vi "laser control with polarimeter feedback.vi"() -> ()   [LabVIEW 2018]
uses:
  <vilib>/DAQmx/read.llb/DAQmx Read (Analog Wfm 1Chan NSamp).vi
  <vilib>/DAQmx/write.llb/DAQmx Write (Analog DBL 1Chan 1Samp).vi
  <vilib>/DAQmx/create/channels.llb/DAQmx Create Channel (AO-Voltage-Basic).vi
  <vilib>/DAQmx/create/channels.llb/DAQmx Create Channel (AI-Voltage-Basic).vi
  <vilib>/DAQmx/configure/timing.llb/DAQmx Timing (Sample Clock).vi
  <vilib>/DAQmx/miscellaneous.llb/DAQmx Fill In Error Info.vi
  <vilib>/ptbypt/NI_PtbyPt.lvlib
panel:
  in  "number of samples per channel":i32=-1
  out "Waveform Chart":dbl(graph)
  in  "stop":bool
  in  "laser voltage":dbl
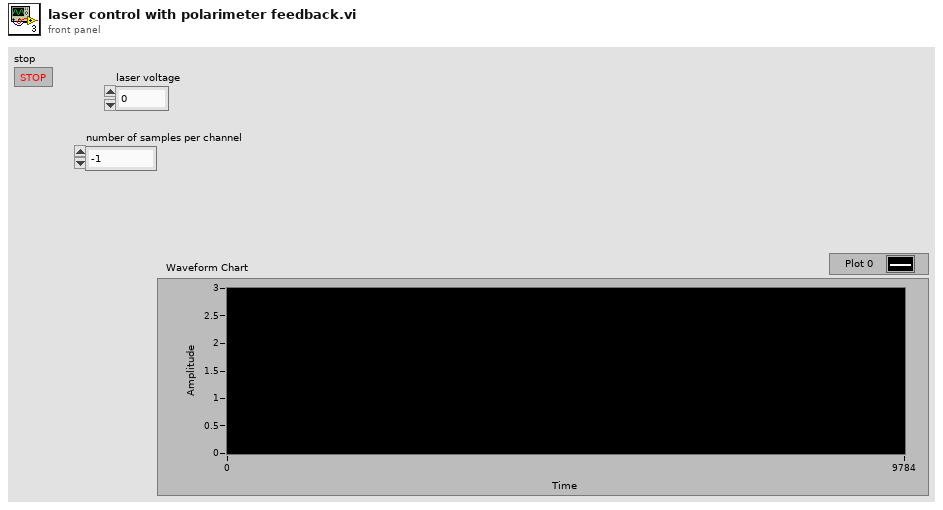
[diagram p1: front panel]
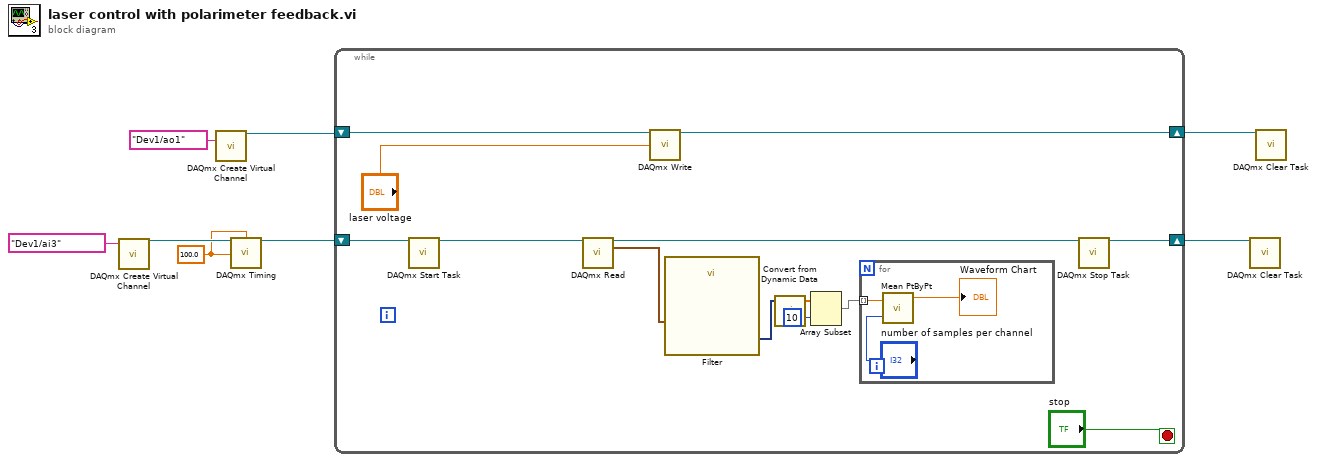
[diagram p0: block diagram]
diagram:
  w1 = 100.0 ("rate")
  n1 = call-poly <vilib>:"DAQmx Create Virtual Channel.vi"("physical channels"=tag "Dev1/ai3") -> ("task out"=w4:refnum<k21>)  [unwired: 13 in, 1 out]
  n2 = call-poly <vilib>:"DAQmx Create Virtual Channel.vi"("physical channels"=tag "Dev1/ao1") -> ("task out"=w6:refnum<k21>)  [unwired: 13 in, 1 out]
  n3 = call-poly <vilib>:"DAQmx Timing.vi"("task/channels in"=w4, "samples per channel"=w1, "rate"=w1) -> ("task out"=w2:refnum<k21>)  [unwired: 11 in, 1 out]
  n4 = while {
    shift-right: [w19] -> w7
    shift-left: w6 -> [w21]
    shift-right: [w14] -> w3
    shift-left: w2 -> [w18]
    stop <- "stop" stop-if-true
    n5 = call <vilib>:"DAQmx Start Task.vi"("task/channels in"=w18) -> ("task out"=w15:refnum<k21>)  [unwired: 13 in, 1 out]
    n6 = call-poly <vilib>:"DAQmx Read.vi"("task/channels in"=w15) -> ("task out"=w20:refnum<k21>, "data"=w10:waveform(dbl))  [unwired: 12 in, 1 out]
    n7 = call-poly <vilib>:"DAQmx Write.vi"("task/channels in"=w21, "data"="laser voltage") -> ("task out"=w19:refnum<k21>)  [unwired: 11 in, 2 out]
    n8 = call "Filter"("Signal"=w10) -> ("Filtered Signal"=w13:dynamicdata)  [unwired: 9 in, 1 out]
    n9 = call "Convert from Dynamic Data"("Dynamic Data Type"=w13) -> ("Array"=w12:dbl[])  [unwired: 3 in]
    n10 = Array Subset(array=w12, index=10) -> (w9:dbl[])  [unwired: 1 in]
    n11 = for {
      tunnel: w9 -> [w22] mode=indexing
      n12 = call <vilib>:"Mean PtByPt.vi"("x"=w22, "sample length"="number of samples per channel") -> ("mean"=→"Waveform Chart":dbl)  [unwired: 2 in, 1 out]
    }
    n13 = call <vilib>:"DAQmx Stop Task.vi"("task/channels in"=w20) -> ("task out"=w14:refnum<k21>)  [unwired: 13 in, 1 out]
  }
  n14 = call <vilib>:"DAQmx Clear Task.vi"("task in"=w3) -> ()  [unwired: 14 in, 1 out]
  n15 = call <vilib>:"DAQmx Clear Task.vi"("task in"=w7) -> ()  [unwired: 14 in, 1 out]
